vi "VI Tree.vi"   [LabVIEW 2011, in "GPT-9000.lvlib"]
doc: "This is the instrument driver for the <INSTRUMENT NAME>. The VI Tree displays all the user-callable VIs of the instrument driver in an organized table."
uses:
  <instrlib>/GPT-9000/GPT-9000.lvlib
panel:
  # "SEE DIAGRAM\nFOR VI TREE."
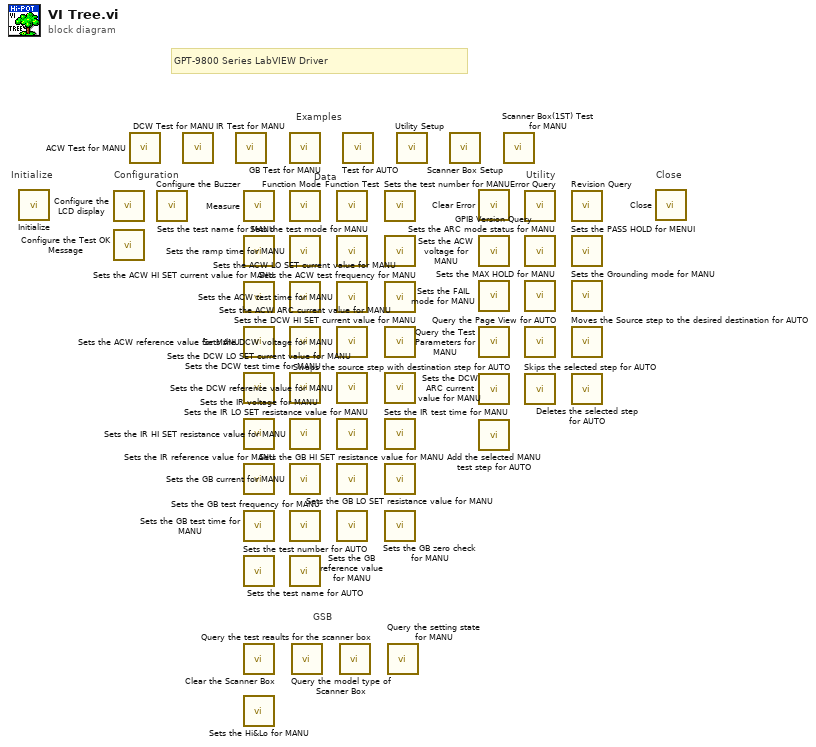
[diagram p0: block diagram]
diagram:
  # "GSB"
  # "Examples"
  # "GPT-9800 Series LabVIEW Driver"
  # "Configuration"
  # "Utility"
  # "Data"
  # "Close"
  # "Initialize"
  n1 = call <instrlib>:"Initialize.vi"() -> ()  [unwired: 8 in, 4 out]
  n2 = call <instrlib>:"Configure the LCD display.vi"() -> ()  [unwired: 8 in, 4 out]
  n3 = call <instrlib>:"Configure the Test OK Message.vi"() -> ()  [unwired: 9 in, 3 out]
  n4 = call <instrlib>:"ACW Test for MANU.vi"() -> ()  [unwired: 10 in, 2 out]
  n5 = call <instrlib>:"Configure the Buzzer.vi"() -> ()  [unwired: 8 in, 4 out]
  n6 = call <instrlib>:"DCW Test for MANU.vi"() -> ()  [unwired: 10 in, 2 out]
  n7 = call <instrlib>:"IR Test for MANU.vi"() -> ()  [unwired: 10 in, 2 out]
  n8 = call <instrlib>:"Measure.vi"() -> ()  [unwired: 12 in, 4 out]
  n9 = call <instrlib>:"Sets the test name for MANU.vi"() -> ()  [unwired: 9 in, 3 out]
  n10 = call <instrlib>:"Sets the ACW HI SET current value for MANU.vi"() -> ()  [unwired: 9 in, 3 out]
  n11 = call <instrlib>:"Sets the ACW reference value for MANU.vi"() -> ()  [unwired: 9 in, 3 out]
  n12 = call <instrlib>:"Sets the DCW LO SET current value for MANU.vi"() -> ()  [unwired: 9 in, 3 out]
  n13 = call <instrlib>:"Sets the IR voltage for MANU.vi"() -> ()  [unwired: 9 in, 3 out]
  n14 = call <instrlib>:"Sets the IR reference value for MANU.vi"() -> ()  [unwired: 9 in, 3 out]
  n15 = call <instrlib>:"Sets the GB test time for MANU.vi"() -> ()  [unwired: 9 in, 3 out]
  n16 = call <instrlib>:"Sets the test number for AUTO.vi"() -> ()  [unwired: 9 in, 3 out]
  n17 = call <instrlib>:"Clear the Scanner Box.vi"() -> ()  [unwired: 10 in, 2 out]
  n18 = call <instrlib>:"Sets the Hi&Lo for MANU.vi"() -> ()  [unwired: 12 in, 4 out]
  n19 = call <instrlib>:"GB Test for MANU.vi"() -> ()  [unwired: 10 in, 2 out]
  n20 = call <instrlib>:"Function Mode.vi"() -> ()  [unwired: 9 in, 3 out]
  n21 = call <instrlib>:"Sets the ramp time for MANU.vi"() -> ()  [unwired: 9 in, 3 out]
  n22 = call <instrlib>:"Sets the ACW LO SET current value for MANU.vi"() -> ()  [unwired: 9 in, 3 out]
  n23 = call <instrlib>:"Sets the ACW ARC current value for MANU.vi"() -> ()  [unwired: 9 in, 3 out]
  n24 = call <instrlib>:"Sets the DCW test time for MANU.vi"() -> ()  [unwired: 9 in, 3 out]
  n25 = call <instrlib>:"Sets the IR HI SET resistance value for MANU.vi"() -> ()  [unwired: 9 in, 3 out]
  n26 = call <instrlib>:"Sets the GB current for MANU.vi"() -> ()  [unwired: 9 in, 3 out]
  n27 = call <instrlib>:"Sets the GB test frequency for MANU.vi"() -> ()  [unwired: 9 in, 3 out]
  n28 = call <instrlib>:"Sets the test name for AUTO.vi"() -> ()  [unwired: 9 in, 3 out]
  n29 = call <instrlib>:"Query the model type of Scanner Box.vi"() -> ()  [unwired: 14 in, 6 out]
  n30 = call <instrlib>:"Function Test.vi"() -> ()  [unwired: 8 in, 3 out]
  n31 = call <instrlib>:"Sets the test mode for MANU.vi"() -> ()  [unwired: 9 in, 3 out]
  n32 = call <instrlib>:"Sets the ACW test time for MANU.vi"() -> ()  [unwired: 9 in, 3 out]
  n33 = call <instrlib>:"Sets the DCW voltage for MANU.vi"() -> ()  [unwired: 9 in, 3 out]
  n34 = call <instrlib>:"Sets the DCW reference value for MANU.vi"() -> ()  [unwired: 9 in, 3 out]
  n35 = call <instrlib>:"Sets the IR LO SET resistance value for MANU.vi"() -> ()  [unwired: 9 in, 3 out]
  n36 = call <instrlib>:"Sets the GB HI SET resistance value for MANU.vi"() -> ()  [unwired: 9 in, 3 out]
  n37 = call <instrlib>:"Sets the GB reference value for MANU.vi"() -> ()  [unwired: 9 in, 3 out]
  n38 = call <instrlib>:"Query the test reaults for the scanner box.vi"() -> ()  [unwired: 14 in, 6 out]
  n39 = call <instrlib>:"Test for AUTO.vi"() -> ()  [unwired: 10 in, 2 out]
  n40 = call <instrlib>:"Sets the test number for MANU.vi"() -> ()  [unwired: 9 in, 3 out]
  n41 = call <instrlib>:"Sets the ACW voltage for MANU.vi"() -> ()  [unwired: 9 in, 3 out]
  n42 = call <instrlib>:"Sets the ACW test frequency for MANU.vi"() -> ()  [unwired: 9 in, 3 out]
  n43 = call <instrlib>:"Sets the DCW HI SET current value for MANU.vi"() -> ()  [unwired: 9 in, 3 out]
  n44 = call <instrlib>:"Sets the DCW ARC current value for MANU.vi"() -> ()  [unwired: 9 in, 3 out]
  n45 = call <instrlib>:"Sets the IR test time for MANU.vi"() -> ()  [unwired: 9 in, 3 out]
  n46 = call <instrlib>:"Sets the GB LO SET resistance value for MANU.vi"() -> ()  [unwired: 8 in, 3 out]
  n47 = call <instrlib>:"Sets the GB zero check for MANU.vi"() -> ()  [unwired: 9 in, 3 out]
  n48 = call <instrlib>:"Query the setting state for MANU.vi"() -> ()  [unwired: 14 in, 6 out]
  n49 = call <instrlib>:"Utility Setup.vi"() -> ()  [unwired: 10 in, 2 out]
  n50 = call <instrlib>:"Scanner Box Setup.vi"() -> ()  [unwired: 10 in, 2 out]
  n51 = call <instrlib>:"Clear Error.vi"() -> ()  [unwired: 10 in, 2 out]
  n52 = call <instrlib>:"GPIB Version Query.vi"() -> ()  [unwired: 9 in, 3 out]
  n53 = call <instrlib>:"Sets the FAIL mode for MANU.vi"() -> ()  [unwired: 9 in, 3 out]
  n54 = call <instrlib>:"Query the Test Parameters for MANU.vi"() -> ()  [unwired: 8 in, 4 out]
  n55 = call <instrlib>:"Swaps the source step with destination step for AUTO.vi"() -> ()  [unwired: 10 in, 2 out]
  n56 = call <instrlib>:"Add the selected MANU test step for AUTO.vi"() -> ()  [unwired: 10 in, 2 out]
  n57 = call <instrlib>:"Scanner Box(1ST) Test for MANU.vi"() -> ()  [unwired: 10 in, 2 out]
  n58 = call <instrlib>:"Error Query.vi"() -> ()  [unwired: 8 in, 4 out]
  n59 = call <instrlib>:"Sets the ARC mode status for MANU.vi"() -> ()  [unwired: 9 in, 3 out]
  n60 = call <instrlib>:"Sets the MAX HOLD for MANU.vi"() -> ()  [unwired: 9 in, 3 out]
  n61 = call <instrlib>:"Query the Page View for AUTO.vi"() -> ()  [unwired: 8 in, 4 out]
  n62 = call <instrlib>:"Skips the selected step for AUTO.vi"() -> ()  [unwired: 10 in, 2 out]
  n63 = call <instrlib>:"Revision Query.vi"() -> ()  [unwired: 8 in, 4 out]
  n64 = call <instrlib>:"Sets the PASS HOLD for MENUI.vi"() -> ()  [unwired: 9 in, 3 out]
  n65 = call <instrlib>:"Sets the Grounding mode for MANU.vi"() -> ()  [unwired: 9 in, 3 out]
  n66 = call <instrlib>:"Moves the Source step to the desired destination for AUTO.vi"() -> ()  [unwired: 10 in, 2 out]
  n67 = call <instrlib>:"Deletes the selected step for AUTO.vi"() -> ()  [unwired: 10 in, 2 out]
  n68 = call <instrlib>:"Close.vi"() -> ()  [unwired: 11 in, 1 out]
